vi "Is Error Responce.vi"(11 "Responce":string) -> (2 "Error Code":i8, 3 "Error?":bool)   [LabVIEW 2017, in "Samwontech TEMP2xxx.lvlib"]
uses:
  <instrlib>/Samwontech TEMP2xxx/Samwontech TEMP2xxx.lvlib
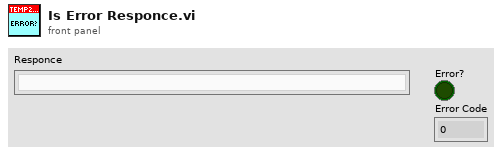
[diagram p1: front panel]
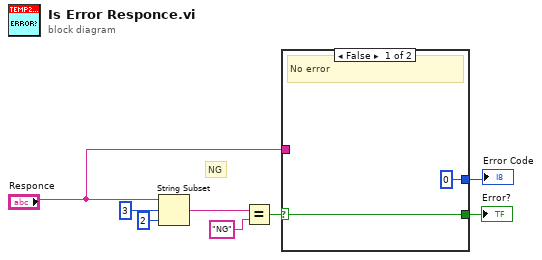
[diagram p0: block diagram]
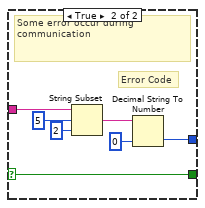
[diagram p2: hidden frame]
diagram:
  # "NG"
  n1 = String Subset(string="Responce", offset (0)=3 ("length (rest)"), length (rest)=2 ("length (rest)")) -> (substring=w5:string)
  n2 = Equal?(x=w5, y="NG") -> (x = y?=w4:bool)
  n3 = case shown="False" w4 {
    selector: w4 -> [w10 w11]
    tunnel: "Responce" -> [_ w15]
    tunnel: [i8 0 w12] -> w1
    tunnel: [w10 w11] -> w2
    frame False {
      # "No error"
    }
    frame True {
      # "Error Code"
      # "Some error occur during communication"
      n4 = String Subset(string=w15, offset (0)=5 ("length (rest)"), length (rest)=2 ("length (rest)")) -> (substring=w13:string)
      n5 = Decimal String To Number(string=w13, default (0L)=i8 0) -> (number=w12:i8)  [unwired: 1 in, 1 out]
    }
  }
  "Error?" <- w2
  "Error Code" <- w1
